vi "Write Direction.vi"(8 "error in (no error)":errorcluster, 10 "Direction":T1, 11 "StatusHistory in":refnum<class "StatusHistory.lvclass">) -> (0 "error out":errorcluster, 3 "StatusHistory out":refnum<class "StatusHistory.lvclass">)   [LabVIEW 2015, in "StatusHistory.lvclass"]
doc: "This property gets or sets the Direction the history is drawn, whether Ascending (Bottom-Up) or Descending (Top-Down).\n<b> </b> <b> </b>\n©2016 Q Software Innovations, LLC (QSI)\nwritten by Quentin Alldredge\nproduced in LabVIEW 2015\n\nsupport@qsoftwareinnovations.com\nwww.qsoftwareinnovations.com\n\nAll rights reserved.\n\nRedistribution and use in source and binary forms, with or without modification, are permitted provided that the following conditions are met:\n\n * Redistributions of source code must retain the above copyright notice, this list of conditions and the following disclaimer.\n * Redistributions in binary form must reproduce the above copyright notice, this list of conditions and the following disclaimer in the documentation and/or other materials provided with the distribution.\n * Neither the name of Q Software Innovations, LLC. nor the names of its contributors may be used to endorse or promote products derived from this software without specific prior written permission.\n\nTHIS SOFTWARE IS PROVIDED BY THE COPYRIGHT HOLDERS AND CONTRIBUTORS \"AS IS\" AND ANY EXPRESS OR IMPLIED WARRANTIES, INCLUDING, BUT NOT LIMITED TO, THE IMPLIED WARRANTIES OF MERCHANTABILITY AND FITNESS FOR A PARTICULAR PURPOSE ARE DISCLAIMED. IN NO EVENT SHALL THE COPYRIGHT OWNER OR CONTRIBUTORS BE LIABLE FOR ANY DIRECT, INDIRECT, INCIDENTAL, SPECIAL, EXEMPLARY, OR CONSEQUENTIAL DAMAGES (INCLUDING, BUT NOT LIMITED TO, PROCUREMENT OF SUBSTITUTE GOODS OR SERVICES; LOSS OF USE, DATA, OR PROFITS; OR BUSINESS INTERRUPTION) HOWEVER CAUSED AND ON ANY THEORY OF LIABILITY, WHETHER IN CONTRACT, STRICT LIABILITY, OR TORT (INCLUDING NEGLIGENCE OR OTHERWISE) ARISING IN ANY WAY OUT OF THE USE OF THIS SOFTWARE, EVEN IF ADVISED OF THE POSSIBILITY OF SUCH DAMAGE."
uses:
  StatusHistory.lvclass
  Direction.ctl
  StatusHistory.lvclass/StatusHistory.ctl
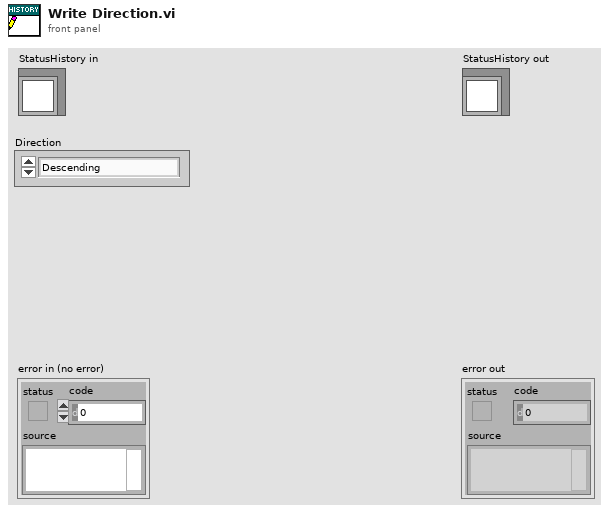
[diagram p1: front panel]
types:
  T1 = typedef "StatusHistory.lvclass/Direction.ctl" = enum16{"Descending", "Ascending"}
  T2 = typedef "StatusHistory.lvclass/State Data.ctl" = cluster{"HistorySize":u32, "Most Recent Color":u32, "Least Recent Color":u32, "Direction":T1, "LockScrolling?":bool}
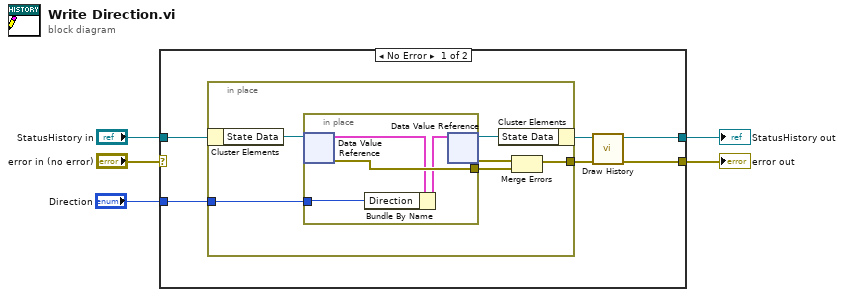
[diagram p0: block diagram]
diagram:
  n1 = case shown="No Error" "error in (no error)" {
    selector: "error in (no error)" -> [_ w22]
    tunnel: [w11 w22] -> w4
    tunnel: [w10 w23] -> w2
    tunnel: "StatusHistory in" -> [w9 w23]
    tunnel: "Direction" -> [w7 _]
    frame No Error {
      n2 = in-place {
        in-place-border: [w13] -> w6
        in-place-border: w7 -> [w12]
        n3 = in-place-cluster #1(w9) -> ("State Data"=w17:refnum<data-value>)
        n4 = in-place {
          in-place-border: [w21] -> w14
          in-place-border: w12 -> [w19]
          n5 = in-place-dvr #2(w17) -> (w18:T2, w21:errorcluster)
          n6 = Bundle By Name(cluster=w18, "Direction"=w19) -> (w20:T2)
          n7 = in-place-dvr #2(w20) -> (w16:refnum<data-value>, w15:errorcluster)
        }
        n8 = in-place-cluster #1("State Data"=w16) -> (w8:refnum<class "StatusHistory.lvclass">)
        n9 = Merge Errors(w15, w14) -> (w13:errorcluster)
      }
      n10 = call "Draw History.vi"("error in (no error)"=w6, "StatusHistory in"=w8) -> ("error out"=w11:errorcluster, "StatusHistory out"=w10:refnum<class "StatusHistory.lvclass">)  [unwired: 8 in]
    }
    frame Error {
    }
  }
  "error out" <- w4
  "StatusHistory out" <- w2
